vi "Set BuildSpec Parameters.vi"(8 "Error In":errorcluster, 11 "Project Sync Tools in":refnum<class "Project Sync Tools.lvclass">) -> (0 "error out":errorcluster, 3 "Project Sync Tools out":refnum<class "Project Sync Tools.lvclass">)   [LabVIEW 2019, in "Project Sync Tools.lvclass"]
uses:
  Project Sync Tools.lvclass
  Project Sync Tools.lvclass/Project Sync Tools.ctl
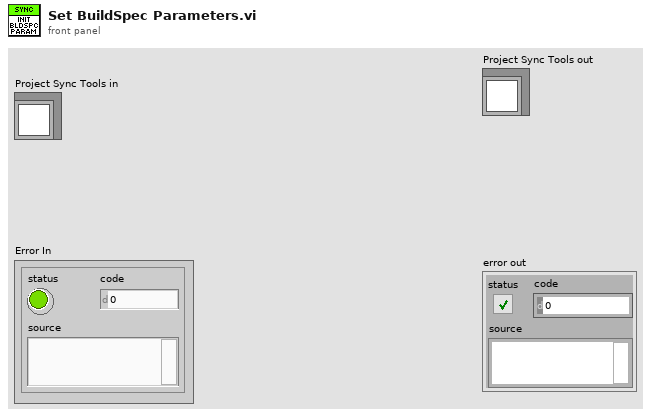
[diagram p1: front panel]
types:
  T1 = typedef "Project Sync Tools.lvclass/BuildSpec Parameters.ctl" = cluster{"BuildSpec Ref":refnum<vi>, "Target Name":string, "Build Spec Name":string, "Tags":string[], "Tag Values":variant[]}
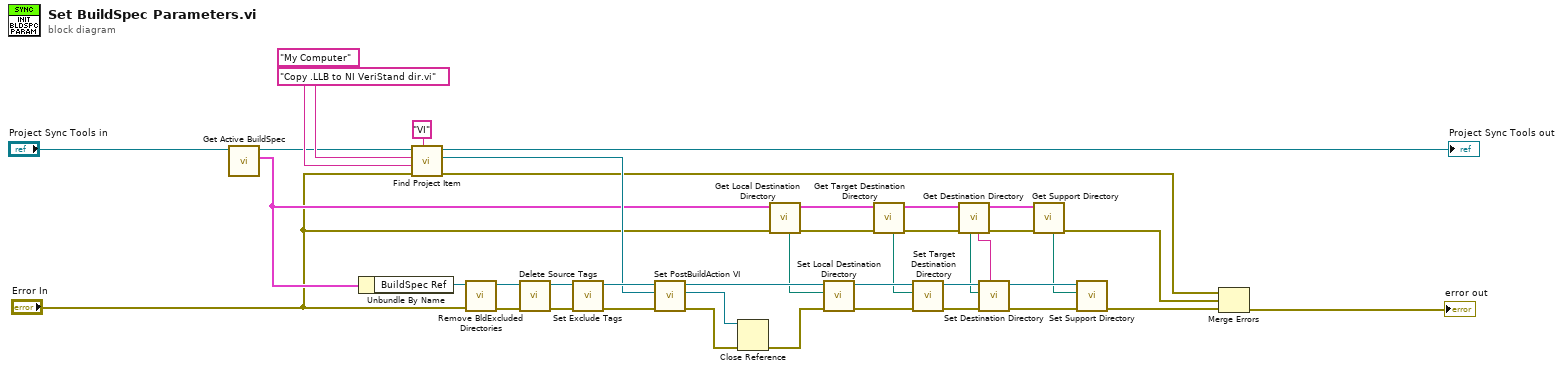
[diagram p0: block diagram]
diagram:
  n1 = call "Get Active BuildSpec.vi"("Project Sync Tools in"="Project Sync Tools in") -> ("Build Spec Parameters"=w7:T1, "Project Sync Tools out"=w8:refnum<class "Project Sync Tools.lvclass">)  [unwired: 9 in]
  n2 = Unbundle By Name(w7) -> ("BuildSpec Ref"=w3:refnum<vi>)
  n3 = call "Find Project Item.vi"("Type"="VI", "error in (no error)"="Error In", "Item Name"="Copy .LLB to NI VeriStand dir.vi" ("Target Item Name"), "Target Name"="My Computer", "Project Sync Tools in"=w8) -> ("error out"=w11:errorcluster, "ProjectItem out"=w25:refnum<vi>, "Project Sync Tools out"=→"Project Sync Tools out":refnum<class "Project Sync Tools.lvclass">)  [unwired: 3 in, 1 out]
  n4 = call "Remove BldExcluded Directories.vi"("error in (no error)"="Error In", "BuildSpec in"=w3) -> ("error out"=w31:errorcluster, "BuildSpec out"=w30:refnum<vi>)  [unwired: 8 in]
  n5 = call "Delete Source Tags.vi"("error in (no error)"=w31, "BuildSpec in"=w30) -> ("error out"=w29:errorcluster, "BuildSpec out"=w28:refnum<vi>)  [unwired: 8 in]
  n6 = call "Set Exclude Tags.vi"("error in (no error)"=w29, "BuildSpec in"=w28) -> ("error out"=w35:errorcluster, "BuildSpec out"=w34:refnum<vi>)  [unwired: 8 in]
  n7 = call "Set PostBuildAction VI.vi"("error in (no error)"=w35, "Project VI in"=w25, "BuildSpec in"=w34) -> ("error out"=w33:errorcluster, "Project VI out"=w23:refnum<vi>, "BuildSpec out"=w32:refnum<vi>)  [unwired: 6 in]
  n8 = Close Reference(reference=w23, error in (no error)=w33) -> (error out=w22:errorcluster)
  n9 = call "Get Local Destination Directory.vi"("error in"="Error In", "Build Spec in"=w7) -> ("error out"=w19:errorcluster, "Build Spec out"=w20:T1, "Local Destination Directory"=w21:path)  [unwired: 7 in]
  n10 = call "Set Local Destination Directory.vi"("error in (no error)"=w22, "Directory path"=w21, "BuildSpec in"=w32) -> ("error out"=w40:errorcluster, "BuildSpec out"=w41:refnum<vi>)  [unwired: 7 in]
  n11 = call "Get Target Destination Directory.vi"("error in"=w19, "Build Spec in"=w20) -> ("error out"=w16:errorcluster, "Build Spec out"=w17:T1, "Target Destination Directory"=w18:path)  [unwired: 7 in]
  n12 = call "Set Target Destination Directory.vi"("error in (no error)"=w40, "Target Destination Directory"=w18, "BuildSpec in"=w41) -> ("error out"=w39:errorcluster, "BuildSpec out"=w36:refnum<vi>)  [unwired: 7 in]
  n13 = call "Get Destination Directory.vi"("error in"=w16, "Build Spec in"=w17) -> ("error out"=w14:errorcluster, "Build Spec out"=w13:T1, "Destination Type"=w1:string, "Target Destination Directory"=w15:path)  [unwired: 6 in]
  n14 = call "Set Destination Directory.vi"("Destination Type"=w1, "error in (no error)"=w39, "Directory Path"=w15, "BuildSpec in"=w36) -> ("error out"=w37:errorcluster, "BuildSpec out"=w38:refnum<vi>)  [unwired: 6 in]
  n15 = call "Get Support Directory.vi"("error in"=w14, "Build Spec in"=w13) -> ("error out"=w5:errorcluster, "Target Destination Directory"=w12:path)  [unwired: 7 in, 1 out]
  n16 = call "Set Support Directory.vi"("error in (no error)"=w37, "Support Directory Path"=w12, "ProjectItem in"=w38) -> ("error out"=w4:errorcluster)  [unwired: 7 in, 1 out]
  n17 = Merge Errors(w11, w5, w4) -> (→"error out":errorcluster)
